vi "from string.vi"(8 "error in":errorcluster, 9 "data":string, 10 "version":string, 11 "UI Reference configuration in":refnum<class "UI Reference configuration.lvclass">) -> (0 "error out":errorcluster, 3 "UI Reference configuration out":refnum<class "UI Reference configuration.lvclass">)   [LabVIEW 2013, in "UI Reference configuration.lvclass"]
doc: "Provides an interface for loading a module configuration from a file or other serialized data source. It is recommended that all children of this class store data in two sets--data required for its own initialization, and any data required for parent initialization--and that each implementation uses the <b>Call Parent Method</b> primitive to de-serialize parent information. As a result, it is expected that every module configuration class calls <b>component configuration.lvclass:From String.vi</b>."
uses:
  UI Reference configuration.lvclass
  <vilib>/NI/Tag Bus Module Framework/module configuration/TBM module configuration.lvclass
  UI Reference configuration.lvclass/UI Reference configuration.ctl
  <vilib>/NI/Tag Bus Module Framework/channel/TBM channel.lvclass
  <vilib>/NI/Tag Bus Module Framework/root configuration/TBM configuration.lvclass
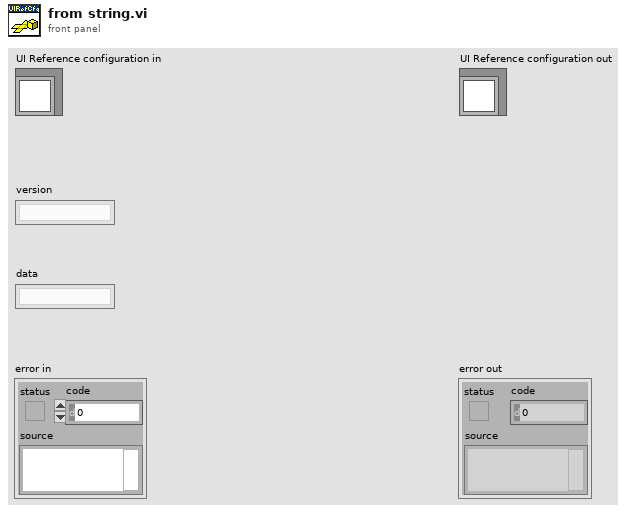
[diagram p1: front panel]
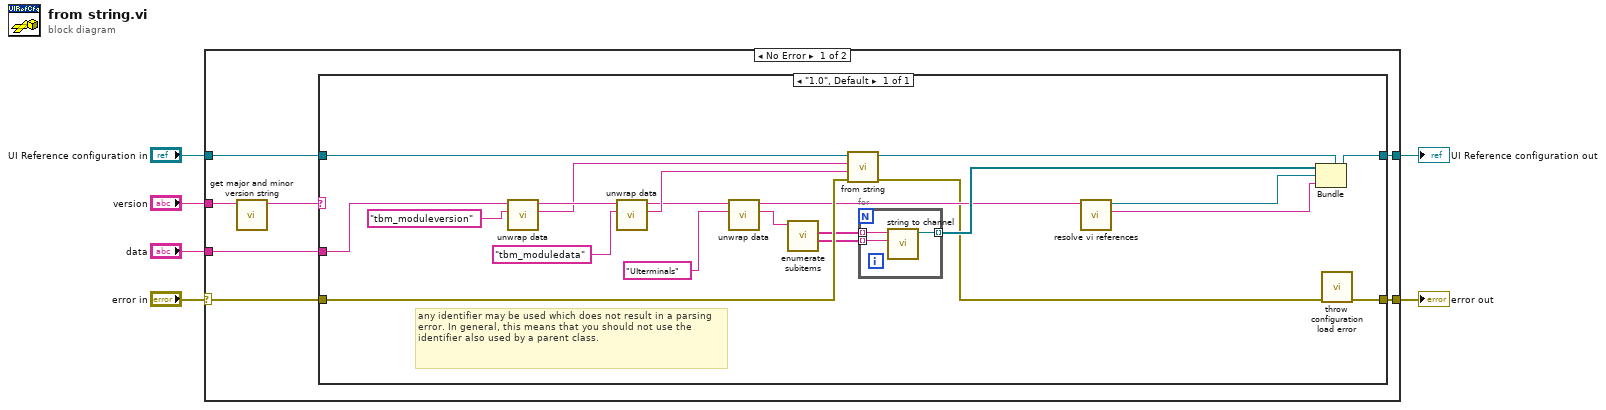
[diagram p0: block diagram]
diagram:
  n1 = case shown="No Error" "error in" {
    selector: "error in" -> [w7 w39]
    tunnel: "data" -> [w13 _]
    tunnel: "UI Reference configuration in" -> [w12 w38]
    tunnel: [w11 w38] -> w5
    tunnel: [w10 w39] -> w4
    tunnel: "version" -> [w9 _]
    frame No Error {
      n2 = call <vilib>:"get major and minor version string.vi"("full version"=w9) -> ("major.minor version"=w8:string)  [unwired: 10 in]
      n3 = case shown="\"1.0\", Default" w8 {
        tunnel: w13 -> [w30]
        tunnel: w7 -> [w29]
        tunnel: w12 -> [w34]
        tunnel: [w24] -> w11
        tunnel: [w32] -> w10
        frame "1.0", Default {
          # "any identifier may be used which does not result in a parsing error. In general, this means that you should not use the identifier also used by a parent class."
          n4 = call <vilib>:"unwrap data.vi"("identifier"="tbm_moduleversion" ("additional identifier"), "data to unwrap"=w30) -> ("unwrapped data"=w25:string, "remaining string"=w31:string)  [unwired: 8 in]
          n5 = call <vilib>:"unwrap data.vi"("identifier"="tbm_moduledata" ("additional identifier"), "data to unwrap"=w31) -> ("unwrapped data"=w27:string, "remaining string"=w23:string)  [unwired: 8 in]
          n6 = call <vilib>:"unwrap data.vi"("identifier"="UIterminals" ("additional identifier"), "data to unwrap"=w23) -> ("unwrapped data"=w21:string, "remaining string"=w17:string)  [unwired: 8 in]
          n7 = call <vilib>:"enumerate subitems.vi"("data to enumerate"=w21) -> ("associated data"=w19:string[], "discovered subitems"=w20:string[])  [unwired: 8 in, 1 out]
          n8 = call-parent "from string.vi"("error in"=w29, "data"=w27, "version"=w25, "module configuration in"=w34) -> ("error out"=w16:errorcluster, "module configuration out"=w33:refnum<class "UI Reference configuration.lvclass">)  [unwired: 6 in]
          n9 = for {
            tunnel: w20 -> [w37] mode=indexing
            tunnel: w19 -> [w36] mode=indexing
            tunnel: [w35] -> w18 mode=indexing
            n10 = call <vilib>:"string to channel.vi"("channel data"=w36, "identifier"=w37) -> ("channel in"=w35:refnum<class "TBM channel.lvclass">)  [unwired: 9 in]
          }
          n11 = call "resolve vi references.vi"("remaining string"=w17) -> ("VI name"=w15:string, "VI out"=w14:refnum<vi>)  [unwired: 9 in]
          n12 = Bundle(cluster=w33, w18, w14, w15) -> (w24:refnum<class "UI Reference configuration.lvclass">)
          n13 = call <vilib>:"throw configuration load error.vi"("error in"=w16) -> ("error out"=w32:errorcluster)  [unwired: 10 in]
        }
      }
    }
    frame Error {
    }
  }
  "error out" <- w4
  "UI Reference configuration out" <- w5
